vi "iRobot Read 16.vi"(11 "stream in":u8[](array[numeric])) -> (0 "value":u16, 3 "stream out":u8[](array[numeric]))   [LabVIEW 2010]
doc: "Read an unsigned 16-bit value from a UART data stream."
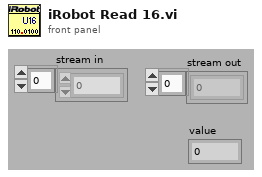
[diagram p1: front panel]
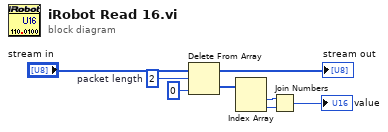
[diagram p0: block diagram]
diagram:
  w6 = 2  # packet length
  n1 = Delete From Array(array="stream in", length=w6, index=0) -> (deleted portion=w5:u8[], array with subset deleted=→"stream out":u8[])
  n2 = Index Array(array=w5) -> (element #1=w2:u8, element #2=w3:u8)  [unwired: 2 in]
  n3 = Join Numbers(hi=w2, lo=w3) -> ((hi.lo)=→"value":u16)
